vi "Exit Screen.vi"(8 "Error In":errorcluster) -> (0 "Error Out":errorcluster, 3 "Status":string)   [LabVIEW 2020]
uses:
  <vilib>/Utility/miscctls.llb/LVPositionTypeDef.ctl
  Control/State - FGV.ctl
  <vilib>/picture/picture.llb/imagedata.ctl
panel:
  out "BG Image":picture
  in  "BG Image old":bool
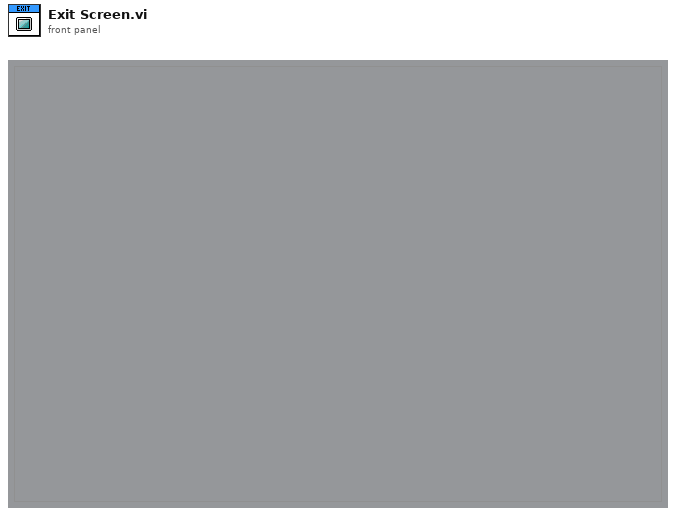
[diagram p1: front panel]
types:
  T1 = typedef "State - FGV.ctl" = enum16{"Write", "Read"}
  T2 = typedef "LVPositionTypeDef.ctl" = cluster{"Left":i32, "Top":i32}
  T3 = typedef "imagedata.ctl" = cluster{"image type":i32, "image depth":i32, "image":u8[], "mask":u8[], "colors":u32[], "Rectangle":cluster{"left":i16, "top":i16, "right":i16, "bottom":i16}}
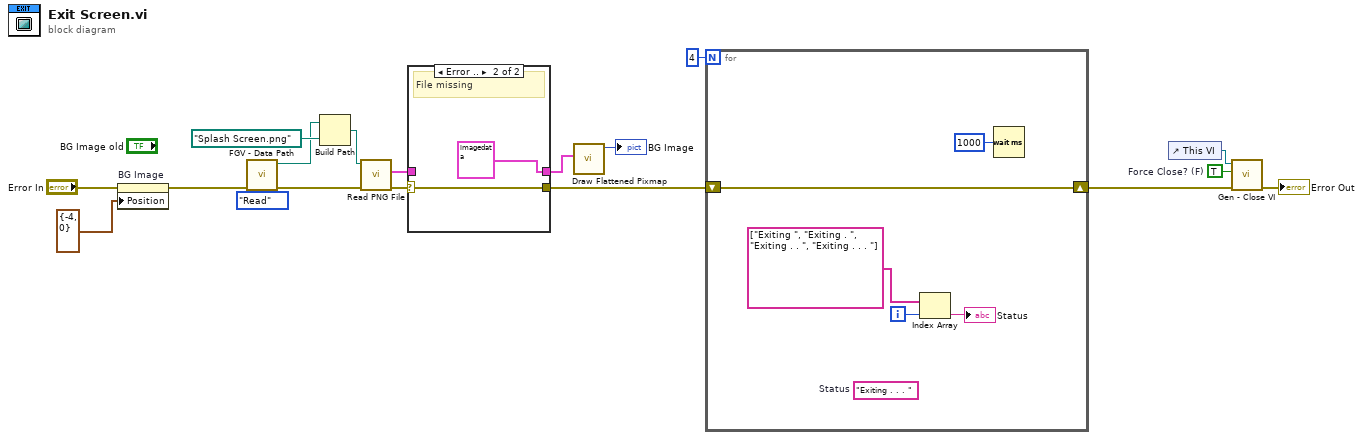
[diagram p0: block diagram]
diagram:
  w1 = TRUE  # Force Close? (F)
  n1 = property on="BG Image" class="Pict"(error in="Error In", "Position"=T2 {"Left"=-4, "Top"=0}) -> (error out=w6:errorcluster)  [unwired: 1 in, 1 out]
  n2 = call "FGV - Data Path.vi"("FGV State"=State_-_FGV."Read", "Error In"=w6) -> ("Error Out"=w7:errorcluster, "Path Out"=w9:path)  [unwired: 8 in]
  n3 = Build Path(base path=w9, name or relative path=path "Splash Screen.png") -> (appended path=w15:path)
  n4 = call <vilib>:"Read PNG File.vi"("error in (no error)"=w7, "path to PNG file"=w15) -> ("error out"=w12:errorcluster, "image data"=w11:T3)  [unwired: 7 in, 1 out]
  n5 = case shown="Error .." w12 {
    selector: w12 -> [w20 w21]
    tunnel: [w20 w21] -> w5
    tunnel: [w19 T3 {"image type"=0, "image depth"=32, "image"=array[1013796 elements], "mask"=array[32184 elements], "colors"=[], "Rectangle"={"left"=0, "top"=0, "right"=567, "bottom"=447}} ("image data")] -> w10
    tunnel: w11 -> [w19 _]
    frame No Error {
    }
    frame Error {
      # "File missing"
    }
  }
  n6 = call <vilib>:"Draw Flattened Pixmap.vi"("image data"=w10) -> ("new picture"=→"BG Image":picture)  [unwired: 8 in]
  n7 = for {
    N: 4 -> [_]
    shift-right: [w27] -> w4
    shift-left: w5 -> [w27]
    i -> [w24]
    (unwired) "Exiting . . . "  # Status
    n8 = Index Array(array=string[] ["Exiting ", "Exiting . ", "Exiting . . ", "Exiting . . . "], index=w24) -> (element=→"Status":string)
    n9 = Wait (ms)(milliseconds to wait=u32 1000) -> ()  [unwired: 1 out]
  }
  n10 = control-ref of="This VI"() -> (w3:refnum<vi>)
  n11 = call "Gen - Close VI.vi"("Error In"=w4, "Force Close? (F)"=w1, "Ref VI"=w3) -> ("Error Out"=→"Error Out":errorcluster)  [unwired: 8 in]
